vi "ChooseClassDialog.vi"() -> (2 "Cancelled":bool, 3 "DMM out":refnum<class "DMM.lvclass">)   [LabVIEW 2012]
doc: "Prompts the user to specify the instrument type, and returns a LabVIEW class reference of the corresponding class. The subsequent steps use dynamic dispatching to call the specified VIs for the selected class"
uses:
  DMM Base/DMM.lvclass
  Simulated DMM/Simulated DMM.lvclass
  PCI-4070/PCI-4070.lvclass
panel:
  in  "OK":bool
  in  "Class":T1(ring)
  # "Select LabVIEW Class Implementation"
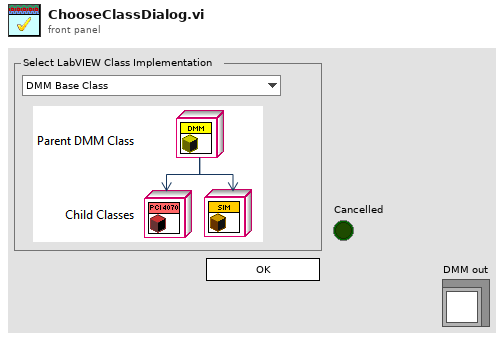
[diagram p1: front panel]
types:
  T1 = enum16{"DMM Base Class", "Simulated DMM", "PCI-4070"}
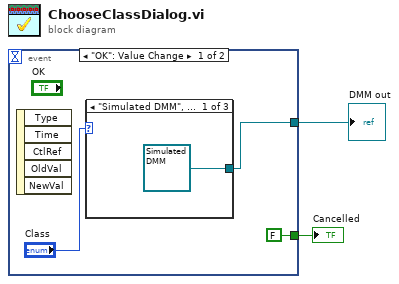
[diagram p0: block diagram]
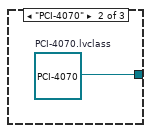
[diagram p2: hidden frame]
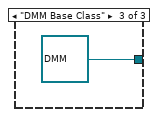
[diagram p3: hidden frame]
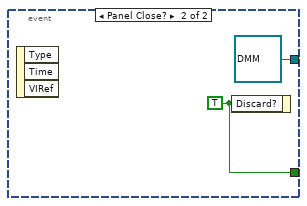
[diagram p4: hidden frame]
diagram:
  n1 = event shown="[0] \"OK\": Value Change" {
    selector: _ -> [_ _]
    dyn-events: _ -> [_ _]
    timeout: _ -> [_ _]
    tunnel: [w5 refnum<class "DMM.lvclass"> refnum ("PCI-4070 out")] -> w2
    tunnel: [FALSE ("Discard?") w10] -> w1
    event "OK": Value Change {
      n2 = event-data() -> ()  [unwired: 1 in, 5 out]
      n3 = case shown="\"Simulated DMM\", Default" "Class" {
        tunnel: [refnum<class "Simulated DMM.lvclass"> refnum ("Simulated DMM.lvclass") w7 refnum<class "DMM.lvclass"> refnum ("PCI-4070 out")] -> w5
        frame "Simulated DMM", Default {
        }
        frame "PCI-4070" {
          w7 = refnum<class "PCI-4070.lvclass"> refnum  # PCI-4070.lvclass
        }
        frame "DMM Base Class" {
        }
      }
    }
    event Panel Close? {
      w10 = TRUE ("Discard?")
      n4 = event-data() -> ()  [unwired: 1 in, 3 out]
      n5 = event-data("Discard?"=w10) -> ()  [unwired: 1 in, 1 out]
    }
  }
  "DMM out" <- w2
  "Cancelled" <- w1
